vi "Polling Stop Core.vi"(8 "Error In":errorcluster, 11 "BNT_ULx-MCSV-DOPWM in":refnum<class "BNT_ULx-MCSV-DOPWM.lvclass">) -> (0 "Error Out":errorcluster, 3 "BNT_ULx-MCSV-DOPWM out":refnum<class "BNT_ULx-MCSV-DOPWM.lvclass">)   [LabVIEW 2020, in "BNT_ULx.lvlib" / "BNT_ULx-MCSV-DOPWM.lvclass"]
doc: "Implement your code to stop polling here."
uses:
  BNT_ULx-MCSV-DOPWM.lvclass
  BNT_ULx-MCSV-DOPWM.lvclass/BNT_ULx-MCSV-DOPWM.ctl
  BNT_ULx-MCSV/BNT_ULx-MCSV.lvclass
  C:/User/Brand/LVP/CSPP/CSPP-Template/Packages/BNT_ULx/BNT_ULx-MCSV/BNT_ULx-MCSV/BNT_ULx-MCSV.lvclass
  C:/User/Brand/LVP/CSPP/CSPP-Template/Packages/CSPP_Core/Actors/CSPP_DeviceActor/CSPP_DeviceActor.lvclass
  C:/User/Brand/LVP/CSPP/CSPP-Template/Packages/CSPP_Core/Actors/CSPP_BaseActor/CSPP_BaseActor.lvclass
  C:/Program Files (x86)/National Instruments/LabVIEW 2020/vi.lib/ActorFramework/Actor/Actor.lvclass
  C:/User/Brand/LVP/CSPP/CSPP-Template/Packages/BNT_ULx/BNT_ULx-MCSV/BNT_ULx-MCSV-DOPWM/BNT_ULx-MCSV-DOPWM.lvclass
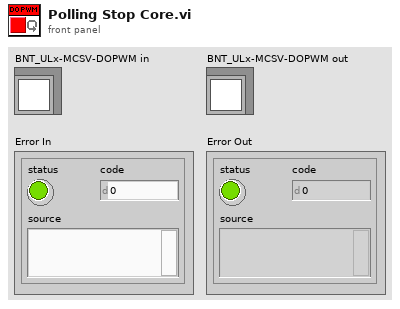
[diagram p1: front panel]
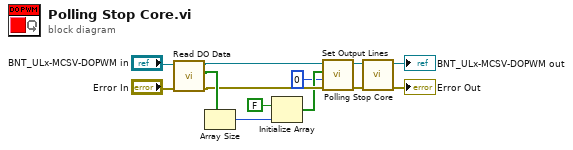
[diagram p0: block diagram]
diagram:
  n1 = call "Read DO Data.vi"("error in (no error)"="Error In", "BNT_DAQmx-MCSV in"="BNT_ULx-MCSV-DOPWM in") -> ("error out"=w3:errorcluster, "DO Data"=w7:bool[], "BNT_DAQmx-MCSV out"=w6:refnum<class "BNT_ULx-MCSV-DOPWM.lvclass">)  [unwired: 7 in]
  n2 = Array Size(array=w7) -> (size(s)=w10:i32)
  n3 = Initialize Array(FALSE, w10) -> (w2:bool[])
  n4 = call "Set Output Lines.vi"("Error In"=w3, "Start Index"=0, "DO Lines"=w2, "BNT_ULx-MCSV in"=w6) -> ("Error Out"=w4:errorcluster, "BNT_ULx-MCSV out"=w5:refnum<class "BNT_ULx-MCSV-DOPWM.lvclass">)  [unwired: 6 in]
  n5 = call-parent "Polling Stop Core.vi"("Error In"=w4, "CSPP_BaseActor in"=w5) -> ("Error Out"=→"Error Out":errorcluster, "CSPP_BaseActor out"=→"BNT_ULx-MCSV-DOPWM out":refnum<class "BNT_ULx-MCSV-DOPWM.lvclass">)  [unwired: 8 in]
